vi "定时启动 (子VI).vi"   [LabVIEW 2016, in "斯坦道CODMn.lvlib"]
types:
  T1 = enum16{"启动测量", "标样核查", "零点核查", "跨度核查", "空白测试", "平行样测试", "加标回收", "空白校准", "标样校准", "初始化（清洗）", "停止测试", "仪器重启", "校时", "模式设置", "测量间隔设置"}
  T2 = cluster{"测量模式":enum16{"水样测量", "标样核查", "零点核查", "跨度核查", "空白测试", "加标回收", "平行样", "校零", "校标"}}
  T3 = cluster{"控制命令":enum16{"启动测量", "标样核查", "零点核查", "跨度核查", "空白测试", "平行样测试", "加标回收", "空白校准", "标样校准", "初始化（清洗）", "停止测试", "仪器重启", "校时", "模式设置", "测量间隔设置"}, "周期设置类型":enum16{"定点启动", "间隔启动"}, "定时功能启用":bool, "定时间隔":dbl, "24H周期设置":bool[], "零点核查时间":u16, "跨度核查时间":u16, "质控频次":enum16{"关闭", "每天", "星期一", "星期二", "星期三", "星期四", "星期五", "星期六", "星期日"}}
  T4 = enum16{"关闭", "每天", "星期一", "星期二", "星期三", "星期四", "星期五", "星期六", "星期日"}
  T5 = typedef "LVDateTimeRec.ctl" = cluster{"秒数的小数部分":dbl, "秒":i32, "分":i32, "时":i32, "日":i32, "月":i32, "年":i32, "天数（周）":i32, "天数（年）":i32, "DST":i32}
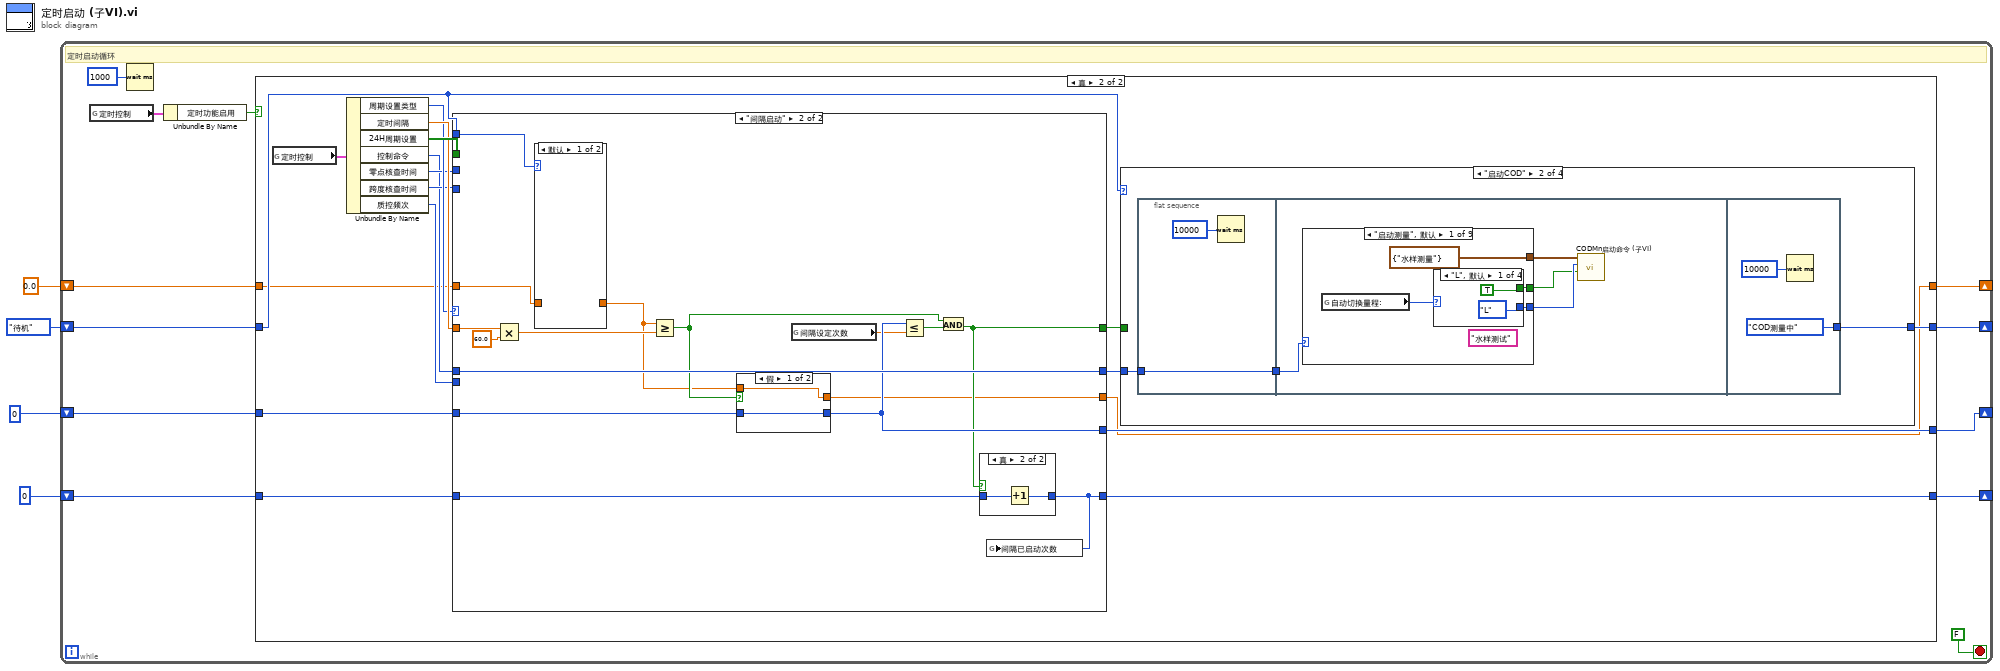
[diagram p0: block diagram]
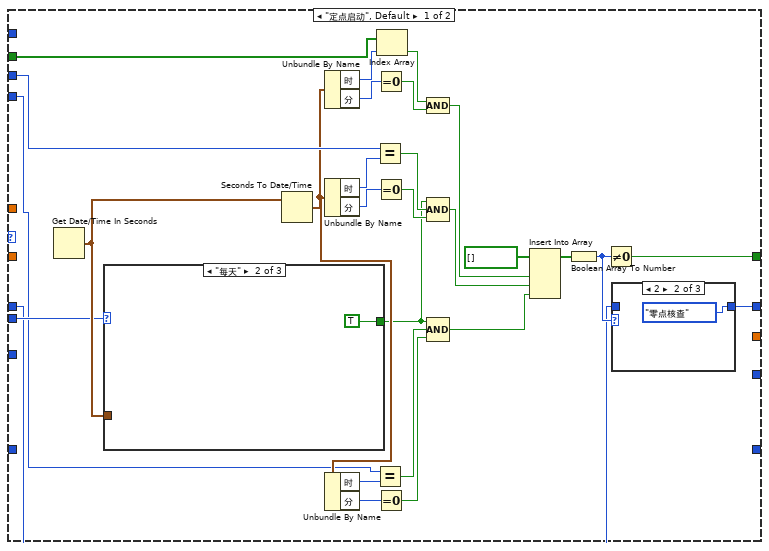
[diagram p3: hidden frame]
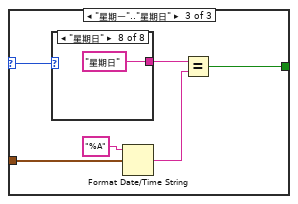
[diagram p5: hidden frame]
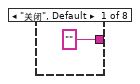
[diagram p6: hidden frame]
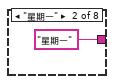
[diagram p7: hidden frame]
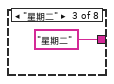
[diagram p8: hidden frame]
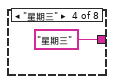
[diagram p9: hidden frame]
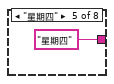
[diagram p10: hidden frame]
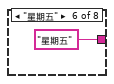
[diagram p11: hidden frame]
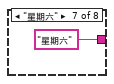
[diagram p12: hidden frame]
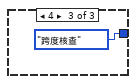
[diagram p14: hidden frame]
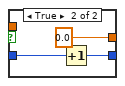
[diagram p16: hidden frame]
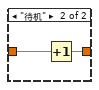
[diagram p17: hidden frame]
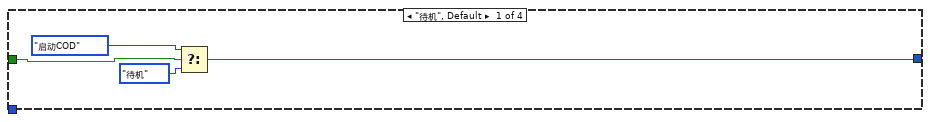
[diagram p18: hidden frame]
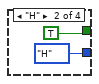
[diagram p19: hidden frame]
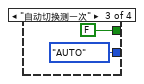
[diagram p20: hidden frame]
diagram:
  n1 = while {
    shift-right: [w15] -> _
    shift-left: enum16{"待机", "启动COD", "COD测量中", "延时"}."待机" -> [w14]
    shift-right: [w9] -> _
    shift-left: 0 -> [w10]
    shift-right: [w7] -> _
    shift-left: 0 -> [w8]
    shift-right: [w5] -> _
    shift-left: 0.0 -> [w6]
    stop <- FALSE stop-if-true
    # "定时启动循环"
    n2 = global read "CODMn断电保存全局变量.vi" "定时控制"() -> (w13:T3)
    n3 = Wait (ms)(milliseconds to wait=u32 1000 ("等待时间（毫秒）")) -> ()  [unwired: 1 out]
    n4 = Unbundle By Name(w13) -> ("定时功能启用"=w12:bool)
    n5 = case shown="真" w12 {
      tunnel: [w17 w35] -> w15
      tunnel: w14 -> [w17 w34]
      tunnel: w10 -> [_ w23]
      tunnel: [_ w22] -> w9
      tunnel: w8 -> [_ w21]
      tunnel: [_ w20] -> w7
      tunnel: w6 -> [_ w19]
      tunnel: [_ w18] -> w5
      frame False {
      }
      frame True {
        n6 = global read "CODMn断电保存全局变量.vi" "定时控制"() -> (w28:T3)
        n7 = Unbundle By Name(w28) -> ("周期设置类型"=w29:enum16{"定点启动", "间隔启动"}, "定时间隔"=w30:dbl, "24H周期设置"=w31:bool[], "控制命令"=w24:T1, "零点核查时间"=w27:u16, "跨度核查时间"=w25:u16, "质控频次"=w26:T4)
        n8 = case shown="\"间隔启动\"" w29 {
          tunnel: w30 -> [_ w96]
          tunnel: w31 -> [w63 _]
          tunnel: w34 -> [_ w97]
          tunnel: [w39 w88] -> w33
          tunnel: w27 -> [w62 _]
          tunnel: w26 -> [w40 _]
          tunnel: w25 -> [w38 _]
          tunnel: w24 -> [w37 w93]
          tunnel: [w36 w93] -> w32
          tunnel: w23 -> [_ w92]
          tunnel: [_ w89] -> w22
          tunnel: w21 -> [_ w87]
          tunnel: [_ w85] -> w20
          tunnel: w19 -> [_ w84]
          tunnel: [_ w83] -> w18
          frame "定点启动", Default {
            n9 = Get Date/Time In Seconds() -> (seconds since 1Jan1904=w58:timestamp)
            n10 = case shown="\"每天\"" w40 {
              selector: w40 -> [_ _ w68]
              tunnel: w58 -> [_ _ w69]
              tunnel: [_ TRUE w65] -> w47
              frame "关闭", Default {
              }
              frame "每天" {
              }
              frame "星期一".."星期日" {
                n11 = case shown="\"星期日\"" w68 {
                  tunnel: ["" ("时间格式字符串(%c)") "星期一" ("时间格式字符串(%c)") "星期二" ("时间格式字符串(%c)") "星期三" ("时间格式字符串(%c)") "星期四" ("时间格式字符串(%c)") "星期五" ("时间格式字符串(%c)") "星期六" ("时间格式字符串(%c)") "星期日" ("时间格式字符串(%c)")] -> w67
                  frame "关闭", Default {
                  }
                  frame "星期一" {
                  }
                  frame "星期二" {
                  }
                  frame "星期三" {
                  }
                  frame "星期四" {
                  }
                  frame "星期五" {
                  }
                  frame "星期六" {
                  }
                  frame "星期日" {
                  }
                }
                n12 = Format Date/Time String(time format string (%c)="%A" ("时间格式字符串(%c)"), seconds (now)=w69) -> (date/time string=w66:string)  [unwired: 1 in]
                n13 = Equal?(x=w67, y=w66) -> (x = y?=w65:bool)
              }
            }
            n14 = Seconds To Date/Time(time stamp (now)=w58) -> (date time rec=w48:T5)  [unwired: 1 in]
            n15 = Unbundle By Name(w48) -> ("时"=w61:i32, "分"=w60:i32)
            n16 = Unbundle By Name(w48) -> ("时"=w55:i32, "分"=w56:i32)
            n17 = Unbundle By Name(w48) -> ("时"=w50:i32, "分"=w49:i32)
            n18 = Equal?(x=w62, y=w55) -> (x = y?=w54:bool)
            n19 = Equal?(x=w38, y=w50) -> (x = y?=w51:bool)
            n20 = Equal To 0?(x=w60) -> (x = 0?=w59:bool)
            n21 = Equal To 0?(x=w56) -> (x = 0?=w53:bool)
            n22 = Equal To 0?(x=w49) -> (x = 0?=w52:bool)
            n23 = Index Array(array=w63, index=w61) -> (element=w57:bool)
            n24 = Compound Arithmetic op=AND ("复合运算")(w57, w59) -> (w45:bool)
            n25 = Compound Arithmetic op=AND ("复合运算")(w47, w54, w53) -> (w44:bool)
            n26 = Compound Arithmetic op=AND ("复合运算")(w47, w51, w52) -> (w43:bool)
            n27 = Insert Into Array(array=bool[] [], new element #1=w45, new element #2=w44, new element #3=w43) -> (w42:bool[])  [unwired: 1 in]
            n28 = Boolean Array To Number(Boolean array=w42) -> (number=w41:u32)
            n29 = Not Equal To 0?(x=w41) -> (x != 0?=w39:bool)
            n30 = case shown="2" w41 {
              tunnel: [w79 T1."零点核查" ("控制命令") T1."跨度核查" ("控制命令")] -> w36
              tunnel: w37 -> [w79 _ _]
              frame 0, Default {
              }
              frame 2 {
              }
              frame 4 {
              }
            }
          }
          frame "间隔启动" {
            n31 = Multiply(x=w96, y=60.0) -> (x*y=w94:dbl)
            n32 = case shown="默认" w97 {
              tunnel: w84 -> [_ w107]
              tunnel: [_ w106] -> w82
              frame Default {
              }
              frame "待机" {
                n33 = Increment(x=w107) -> (x+1=w106:dbl)
              }
            }
            n34 = Greater Or Equal?(x=w82, y=w94) -> (x >= y?=w90:bool)
            n35 = case shown="假" w90 {
              tunnel: w92 -> [w102 w105]
              tunnel: [w102 w104] -> w89
              tunnel: [w101 0.0] -> w83
              tunnel: w82 -> [w101 _]
              frame False {
              }
              frame True {
                n36 = Increment(x=w105) -> (x+1=w104:i32)
              }
            }
            n37 = global read "CODMn断电保存全局变量.vi" "间隔设定次数"() -> (w86:dbl)
            n38 = Less Or Equal?(x=w89, y=w86) -> (x <= y?=w91:bool)
            n39 = And(x=w90, y=w91) -> (x .and. y?=w88:bool)
            n40 = case shown="真" w88 {
              tunnel: w87 -> [w98 w100]
              tunnel: [w98 w99] -> w85
              frame False {
              }
              frame True {
                n41 = Increment(x=w100) -> (x+1=w99:i32)
              }
            }
            n42 = global write "CODMn断电保存全局变量.vi" "间隔已启动次数"(w85) -> ()
          }
        }
        n43 = case shown="\"启动COD\"" w34 {
          tunnel: [w108 w114 w156 enum16{"待机", "启动COD", "COD测量中", "延时"}."待机"] -> w35
          tunnel: w33 -> [w111 _ _ _]
          tunnel: w32 -> [_ w112 _ _]
          frame "待机", Default {
            n44 = Select(t=enum16{"待机", "启动COD", "COD测量中", "延时"}."启动COD", s=w111, f=enum16{"待机", "启动COD", "COD测量中", "延时"}."待机") -> (s? t:f=w108:enum16{"待机", "启动COD", "COD测量中", "延时"})
          }
          frame "启动COD" {
            n45 = flat-sequence {
              tunnel: w112 -> [w116]
              tunnel: [w116] -> w113
              tunnel: w113 -> [w120]
              tunnel: [enum16{"待机", "启动COD", "COD测量中", "延时"}."COD测量中"] -> w114
              frame #0 {
                n46 = Wait (ms)(milliseconds to wait=u32 10000 ("等待时间（毫秒）")) -> ()  [unwired: 1 out]
              }
              frame #1 {
                n47 = case shown="\"启动测量\", 默认" w120 {
                  tunnel: [T2 {"测量模式"=enum."水样测量"} ("启动测量模式") T2 {"测量模式"=enum."标样核查"} ("启动测量模式") T2 {"测量模式"=enum."空白测试"} ("启动测量模式") T2 {"测量模式"=enum."跨度核查"} ("启动测量模式") T2 {"测量模式"=enum."加标回收"} ("启动测量模式") T2 {"测量模式"=enum."平行样"} ("启动测量模式") T2 {"测量模式"=enum."校零"} ("启动测量模式") T2 {"测量模式"=enum."校标"} ("启动测量模式") T2 {"测量模式"=enum."零点核查"} ("启动测量模式")] -> w119
                  tunnel: [w123 w133 enum32{"H", "L", "AUTO"}."L" ("CODMn跨度量程选择") w137 enum32{"H", "L", "AUTO"}."AUTO" ("CODMn跨度量程选择") enum32{"H", "L", "AUTO"}."AUTO" ("CODMn跨度量程选择") enum32{"H", "L", "AUTO"}."L" ("CODMn跨度量程选择") enum32{"H", "L", "AUTO"}."AUTO" ("CODMn跨度量程选择") w147] -> w118
                  tunnel: [w122 _ _ _ _ _ _ _ _] -> w117
                  frame "启动测量", Default {
                    (unwired) "水样测试" ("测量模式")
                    n48 = global read "CODMn断电保存全局变量.vi" "自动切换量程:"() -> (w121:enum16{"L", "H", "自动切换测一次", "自动切换测两次"})
                    n49 = case shown="\"L\", 默认" w121 {
                      tunnel: [enum32{"H", "L", "AUTO"}."L" ("CODMn跨度量程选择") enum32{"H", "L", "AUTO"}."H" ("CODMn跨度量程选择") enum32{"H", "L", "AUTO"}."AUTO" ("CODMn跨度量程选择") enum32{"H", "L", "AUTO"}."AUTO" ("CODMn跨度量程选择")] -> w123
                      tunnel: [TRUE TRUE FALSE FALSE] -> w122
                      frame "L", Default {
                      }
                      frame "H" {
                      }
                      frame "自动切换测一次" {
                      }
                      frame "自动切换测两次" {
                      }
                    }
                  }
                  frame "标样核查" {
                    (unwired) "标样核查" ("测量模式")
                    n50 = global read "CODMn断电保存全局变量.vi" "标样核查量程选择"() -> (w133:enum32{"H", "L", "AUTO"})
                  }
                  frame "空白测试" {
                    (unwired) "空白测试" ("测量模式")
                  }
                  frame "跨度核查" {
                    (unwired) "跨度核查" ("测量模式")
                    n51 = global read "CODMn断电保存全局变量.vi" "CODMn跨度量程选择"() -> (w137:enum32{"H", "L", "AUTO"})
                  }
                  frame "加标回收" {
                    (unwired) "加标回收" ("测量模式")
                  }
                  frame "平行样测试" {
                    (unwired) "平行样" ("测量模式")
                  }
                  frame "空白校准" {
                  }
                  frame "标样校准" {
                    (unwired) "校标" ("测量模式")
                  }
                  frame "零点核查" {
                    (unwired) "零点核查" ("测量模式")
                    n52 = global read "CODMn断电保存全局变量.vi" "零点核查量程选择"() -> (w147:enum32{"H", "L", "AUTO"})
                  }
                }
                n53 = call "CODMn启动命令 (子VI).vi"("强制切换"=w117, "CODMn量程切换"=w118, "启动测量模式"=w119) -> ()  [unwired: 9 in]
              }
              frame #2 {
                n54 = Wait (ms)(milliseconds to wait=u32 10000 ("等待时间（毫秒）")) -> ()  [unwired: 1 out]
              }
            }
          }
          frame "COD测量中" {
            n55 = global read "运行时序全局变量.vi" "多列列表框"() -> (w155:i32)
            n56 = Equal?(x=w155, y=0) -> (x = y?=w153:bool)
            n57 = Select(t=enum16{"待机", "启动COD", "COD测量中", "延时"}."延时", s=w153, f=enum16{"待机", "启动COD", "COD测量中", "延时"}."COD测量中") -> (s? t:f=w156:enum16{"待机", "启动COD", "COD测量中", "延时"})
          }
          frame "延时" {
            n58 = Wait (ms)(milliseconds to wait=u32 5000 ("等待时间（毫秒）")) -> ()  [unwired: 1 out]
          }
        }
      }
    }
  }
